vi "Read server context.vi"(11 "lvlibretls server listener in":refnum<class "lvlibretls server listener.lvclass">) -> (2 "server context":u64, 3 "lvlibretls server listener out":refnum<class "lvlibretls server listener.lvclass">)   [LabVIEW 2016, in "lvlibretls server listener.lvclass"]
uses:
  lvlibretls server listener.lvclass
  lvlibretls server listener.lvclass/lvlibretls server listener.ctl
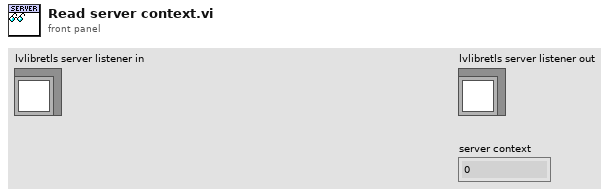
[diagram p1: front panel]
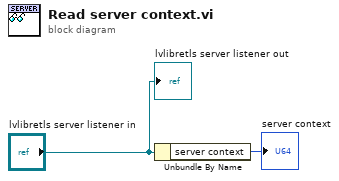
[diagram p0: block diagram]
diagram:
  n1 = Unbundle By Name("lvlibretls server listener in") -> ("server context"=→"server context":u64)
  "lvlibretls server listener out" <- "lvlibretls server listener in"
